vi "_IRR_mkpk.vi"(0 "Bias_LO_equip":T4={"Node address"=19, "CAN Interface"="CAN0", "Cartridge band"=10, "Slave Node in"={"Address"=19, "Serial Number"=[16, -88, -112, 75, 1, 8, 0, 24]}, "ObjHandle out"=93192256, "POL"=0, "sb"=1, "GPIB_SM (SIS S,V)"="24", "GPIB_DMM (SIS I)"="22", "GPIB_SM (MAG I) "="25", "GPIB_SG(LO)"="19", "GPIB_PW (PAMP) "="6", "GPIB_TMP1(8ch)"="12", "GPIB_TMP2(2ch)  "="13", "WCA_avg"=10, "Rsen"=10.0, "BiasModule"=1, "LOModule "=2, "WCA_LO_FREQ_SET"={"YTO Low freq. [GHz]"=14.66, "YTO High freq. [GHz]"=17.5, "Kvco"=1, "Lock Pol."=0, "SET LO FREQ"=88.77778, "Multiplier"=6.0, "YTO (HEX)"=197, "YTO ( FREQ)"=14.796625, "NULL PLL INTEGRATOR"=FALSE}} {"WCA_LO_FREQ_SET"."YTO ( FREQ)" min=25 max=150 step=0.0001 format="%.3f"; "WCA_LO_FREQ_SET"."Multiplier" min=3 max=6 step=3; "WCA_LO_FREQ_SET"."SET LO FREQ" min=25 max=150 step=0.0001 format="%.3f"; "WCA_LO_FREQ_SET"."Lock Pol." items=["Lower", "Upper"]; "WCA_LO_FREQ_SET"."Kvco" items=["7.5MHz/V", "15MHz/V"]; "WCA_LO_FREQ_SET"."YTO High freq. [GHz]" format="%.3f"; "WCA_LO_FREQ_SET"."YTO Low freq. [GHz]" format="%.3f"; "LOModule" items=["Manual Gunn+PAMP"=0, "PLL GUNN+PAMP"=5, "B10Lab LO"=1, "WCA LO"=2, ""=3, "YIG発信器"=4, "none"=99]; "BiasModule" items=["B10Lab Bias"=0, "WCA BiasModule"=1, "none"=99]; "Slave Node in"."Serial Number" format="%.0x"; "Slave Node in"."Address" format="%.0x"; "Cartridge band" max=10 step=1; "Node address" format="%.0x"}, 1 "Control":T8={"GPIB_ATT"="28", "6501Dev#"=1, "GPIB_SP"="18", "GPIB_PM"="13", "GPIB_DSA"="11", "GPIB_DMM (TPD)"="23", "GPIB_MPI"="COM9", "mortor設定"=[{"Axis"=0, "ID"=0, "HIspeed"=200.0, "LOspeed"=100.0, "ACCEL(ms)"=100.0, "Sratio"=50.0, "フリーラン\n"=FALSE, "文字列"="DSB HOT/COLD"}, {"Axis"=1, "ID"=0, "HIspeed"=4.0, "LOspeed"=4.0, "ACCEL(ms)"=100.0, "Sratio"=50.0, "フリーラン\n"=TRUE, "文字列"="SubMM Att"}, {"Axis"=0, "ID"=0, "HIspeed"=200.0, "LOspeed"=100.0, "ACCEL(ms)"=100.0, "Sratio"=50.0, "フリーラン\n"=FALSE, "文字列"="MPI Port1"}, {"Axis"=1, "ID"=0, "HIspeed"=200.0, "LOspeed"=100.0, "ACCEL(ms)"=100.0, "Sratio"=50.0, "フリーラン\n"=FALSE, "文字列"="MPI Port2"}, {"Axis"=1, "ID"=0, "HIspeed"=200.0, "LOspeed"=100.0, "ACCEL(ms)"=100.0, "Sratio"=50.0, "フリーラン\n"=TRUE, "文字列"="gainComp"}], "DATAパス"=path "C:/Documents and Settings/band10/デスクトップ/data/cartridge/CCA03/CCA-03-13/110831_etc", "mixer param file "=path "Z:/band10/Labview_ALMA/MIX95/test", "comment"="xttest", "ColdCarts"="003601", "Th"=299.0, "Tc"=77.0, "Set_SIS_volt"=2.1, "Offset"=0.0, "control"=0, "FreqLO"=799.0, "Set_Mag_Cur"=13.664233576642335, "MPI offset(mm)"=23.152, "HOT/COLD"=0} {"HOT/COLD" items=["DSB", "SBR (Cart.)", "GainComp", "SBR (MIX)"]; "control" items=["CLOSE LOOP", "OPEN LOOP", "Not Control"]}, 2 "CrossTalk_mkpk":T7={"save"=TRUE, "file_name"="xtk_799.00_120_xttest.csv", "IF start"=4.0, "IF stop"=12.0, "IF step"=1.0}, 3 "PAV配列":cluster{"VD":dbl, "VG ":dbl, "文字列":string}[](array[cluster])=[{"VD"=0.0, "VG "=-0.04, "文字列"="WCA P0"}, {"VD"=0.0, "VG "=-0.04, "文字列"="WCA P1"}, {"VD"=1.75, "VG "=2.1, "文字列"="B10 PAMP"}] {"VG" min=-1.0 max=4.0; "VD" min=0.0 max=2.5}, 4 "_LO_P_OPT":T3={"範囲配列"=[{"Start"=1.0, "Stop"=3.5, "Step"=0.01, "ｂｙ"="NEL VG"}, {"Start"=40.0, "Stop"=75.0, "Step"=1.0, "ｂｙ"="Motor"}, {"Start"=1.0, "Stop"=2.5, "Step"=0.1, "ｂｙ"="WCA VD"}], "Optimize"=0, "file_name"="LP_914.0_Tmin_100519.csv", "Save?"=FALSE, "measure"=2, "current(uA)"=60.0, "wait(ms)"=0, "IFfrq(GHz)"=8.0, "aveg"=10, "SISparam option"=2} {"SISparam option" items=["Volt and Current", "Volt only"]; "measure" items=["Pmax (only HOT)", "Tmin (HOT/COLD)", "C current"]; "Optimize" items=["Sweep", "黄金分割"]; "範囲配列"."Step" format="%.2f"; "範囲配列"."Stop" format="%.2f"; "範囲配列"."Start" format="%.2f"}) -> (7 "LOPopt P0":string="LOPt,799.00,1.46,1.88,38.10,0.00,0.00,0.00,2.10,,WCA,0.003815,4.013062,-0.021667,  1.030579,172.775269,-0.025177,")   [LabVIEW 2012]
uses:
  <vilib>/express/express arith-compare/Formula/XNode/ExpressFormulaBlockNode.xnode
panel:
  out "結果":string="4.000015,-97.540000,-93.196000,  -9.974000,-47.367000,-107.514000, -6.485000,-40.957000,-99.681000 , LOPt,799.00,1.46,1.88,38.19,0.00,0.00,0.00,2.19,,WCA,0.003662,3.952026,-0.022125,  1.031342,172.851562,-0.025787, ,LOPt,799.00,1.90,1.89,41.31,0.00,0.00,0.00,0.31,,WCA,1.335449,186.492920,-0.022125,  0.001831,3.158569,-0.025787, \n5.000041,-92.917000,-98.660000,  -10.003000,-45.366000,-102.920000, -7.055000,-44.960000,-105.715000 , LOPt,799.00,1.46,1.88,36.93,0.00,0.00,0.00,0.93,,WCA,0.003510,4.043579,-0.022736,  1.030426,172.744751,-0.025635, ,LOPt,799.00,1.90,1.90,41.12,0.00,0.00,0.00,0.12,,WCA,1.335754,186.691284,-0.021820,  0.001984,3.265381,-0.025330, \n6.000013,-94.024000,-94.568000,  -8.711000,-43.164000,-102.735000, -5.761000,-42.975000,-100.329000 , LOPt,799.00,1.46,1.87,37.45,0.00,0.00,0.00,1.45,,WCA,0.003510,3.936768,-0.022278,  1.030579,172.760010,-0.025940, ,LOPt,799.00,1.90,1.89,41.11,0.00,0.00,0.00,0.11,,WCA,1.336365,186.798096,-0.022736,  0.001831,3.173828,-0.025940, \n"
  out "XYグラフ":cluster{dbl[], dbl[]}[](graph)=[{[4.000015156, 5.000041231, 6.000013312], [-97.53999999999999, -92.917, -94.024]}, {[4.000015156, 5.000041231, 6.000013312], [-93.196, -98.66, -94.568]}]
  out "LOPopt P1":string="LOPt,799.00,1.90,1.89,41.11,0.00,0.00,0.00,0.11,,WCA,1.336365,186.798096,-0.022736,  0.001831,3.173828,-0.025940,"
  out "crossTK P1":dbl=-100.329 format="%#_6p"
  out "xpol P1":dbl=-42.975 format="%#_6p"
  out "copol P1":dbl=-5.761 format="%#_6p"
  in  "SP_set":T1={"start(GHz)"=3.5, "stop(GHz) "=12.5, "BW(MHz)"=0.0001, "VBW(Hz)"=30.0, "ref(dBm)"=0.0, "log(dB)"=15.0, "AVEG"=30, "AVEG ON/OFF"=FALSE, "Auto Align ON/OFF"=FALSE, "GPIB"="18", "point"=801}
  in  "IFBOX":T2={" Output"=1, "YIG Fc(GHz)"=4.0, " Filter"=3, "Input"=1} {"Input" items=["1:Pol 0"=1, "2:Pol 1"=2, "3:dummy"=3, "4:NoiseSource"=4]; "Filter" items=["1:YIG"=1, "2:direct"=2, "3:4-12BPF"=3, "4:direct 4-12BPF"=4]; "Output" items=["1:Speana"=1, "2:PowerMeter"=2, "3:dummy"=3, "4:TPD"=4]}
  in  "RF":T5={"RF(GHz)"=800.0, "mm_multi(4or6)"=6.0, "SGPOUT(dBm)"=10.0, "SGGPIB"="29", "PAMP GPIB"="6", "VD (V)"=1.7, "VG (V)"=2.2, "multi (V)"=8.0} {"multi (V)" min=0.0 max=15.0 step=0.5; "VG (V)" min=0.0 max=4.0 step=0.1; "VD (V)" min=0.0 max=1.85 step=0.1}
  out "crossTK P0":dbl=-102.735 format="%#_6p"
  out "xpol P0":dbl=-43.164 format="%#_6p"
  out "copol P0":dbl=-8.711 format="%#_6p"
  out "frq":dbl=6.000013312 format="%#_6p"
  in  "SIS_Deflux_heater":T6={"ON開始時間（mｓ）"=3000.0, "ON継続時間（mｓ）"=1000.0, "測定終了時間（mｓ）"=60000.0, "SIS Volt（mV)"=0.5, "GPIB_PW (SISHeater) "="3", "SAVE"=TRUE}
  out "初期時間（s）":dbl=3379641043.615625
  # "LO freq. [GHz]"
  # "YTO LOW\n/High Freq."
  # "ZERO Intgrtr"
  # "Node Address"
  # "Serial Number"
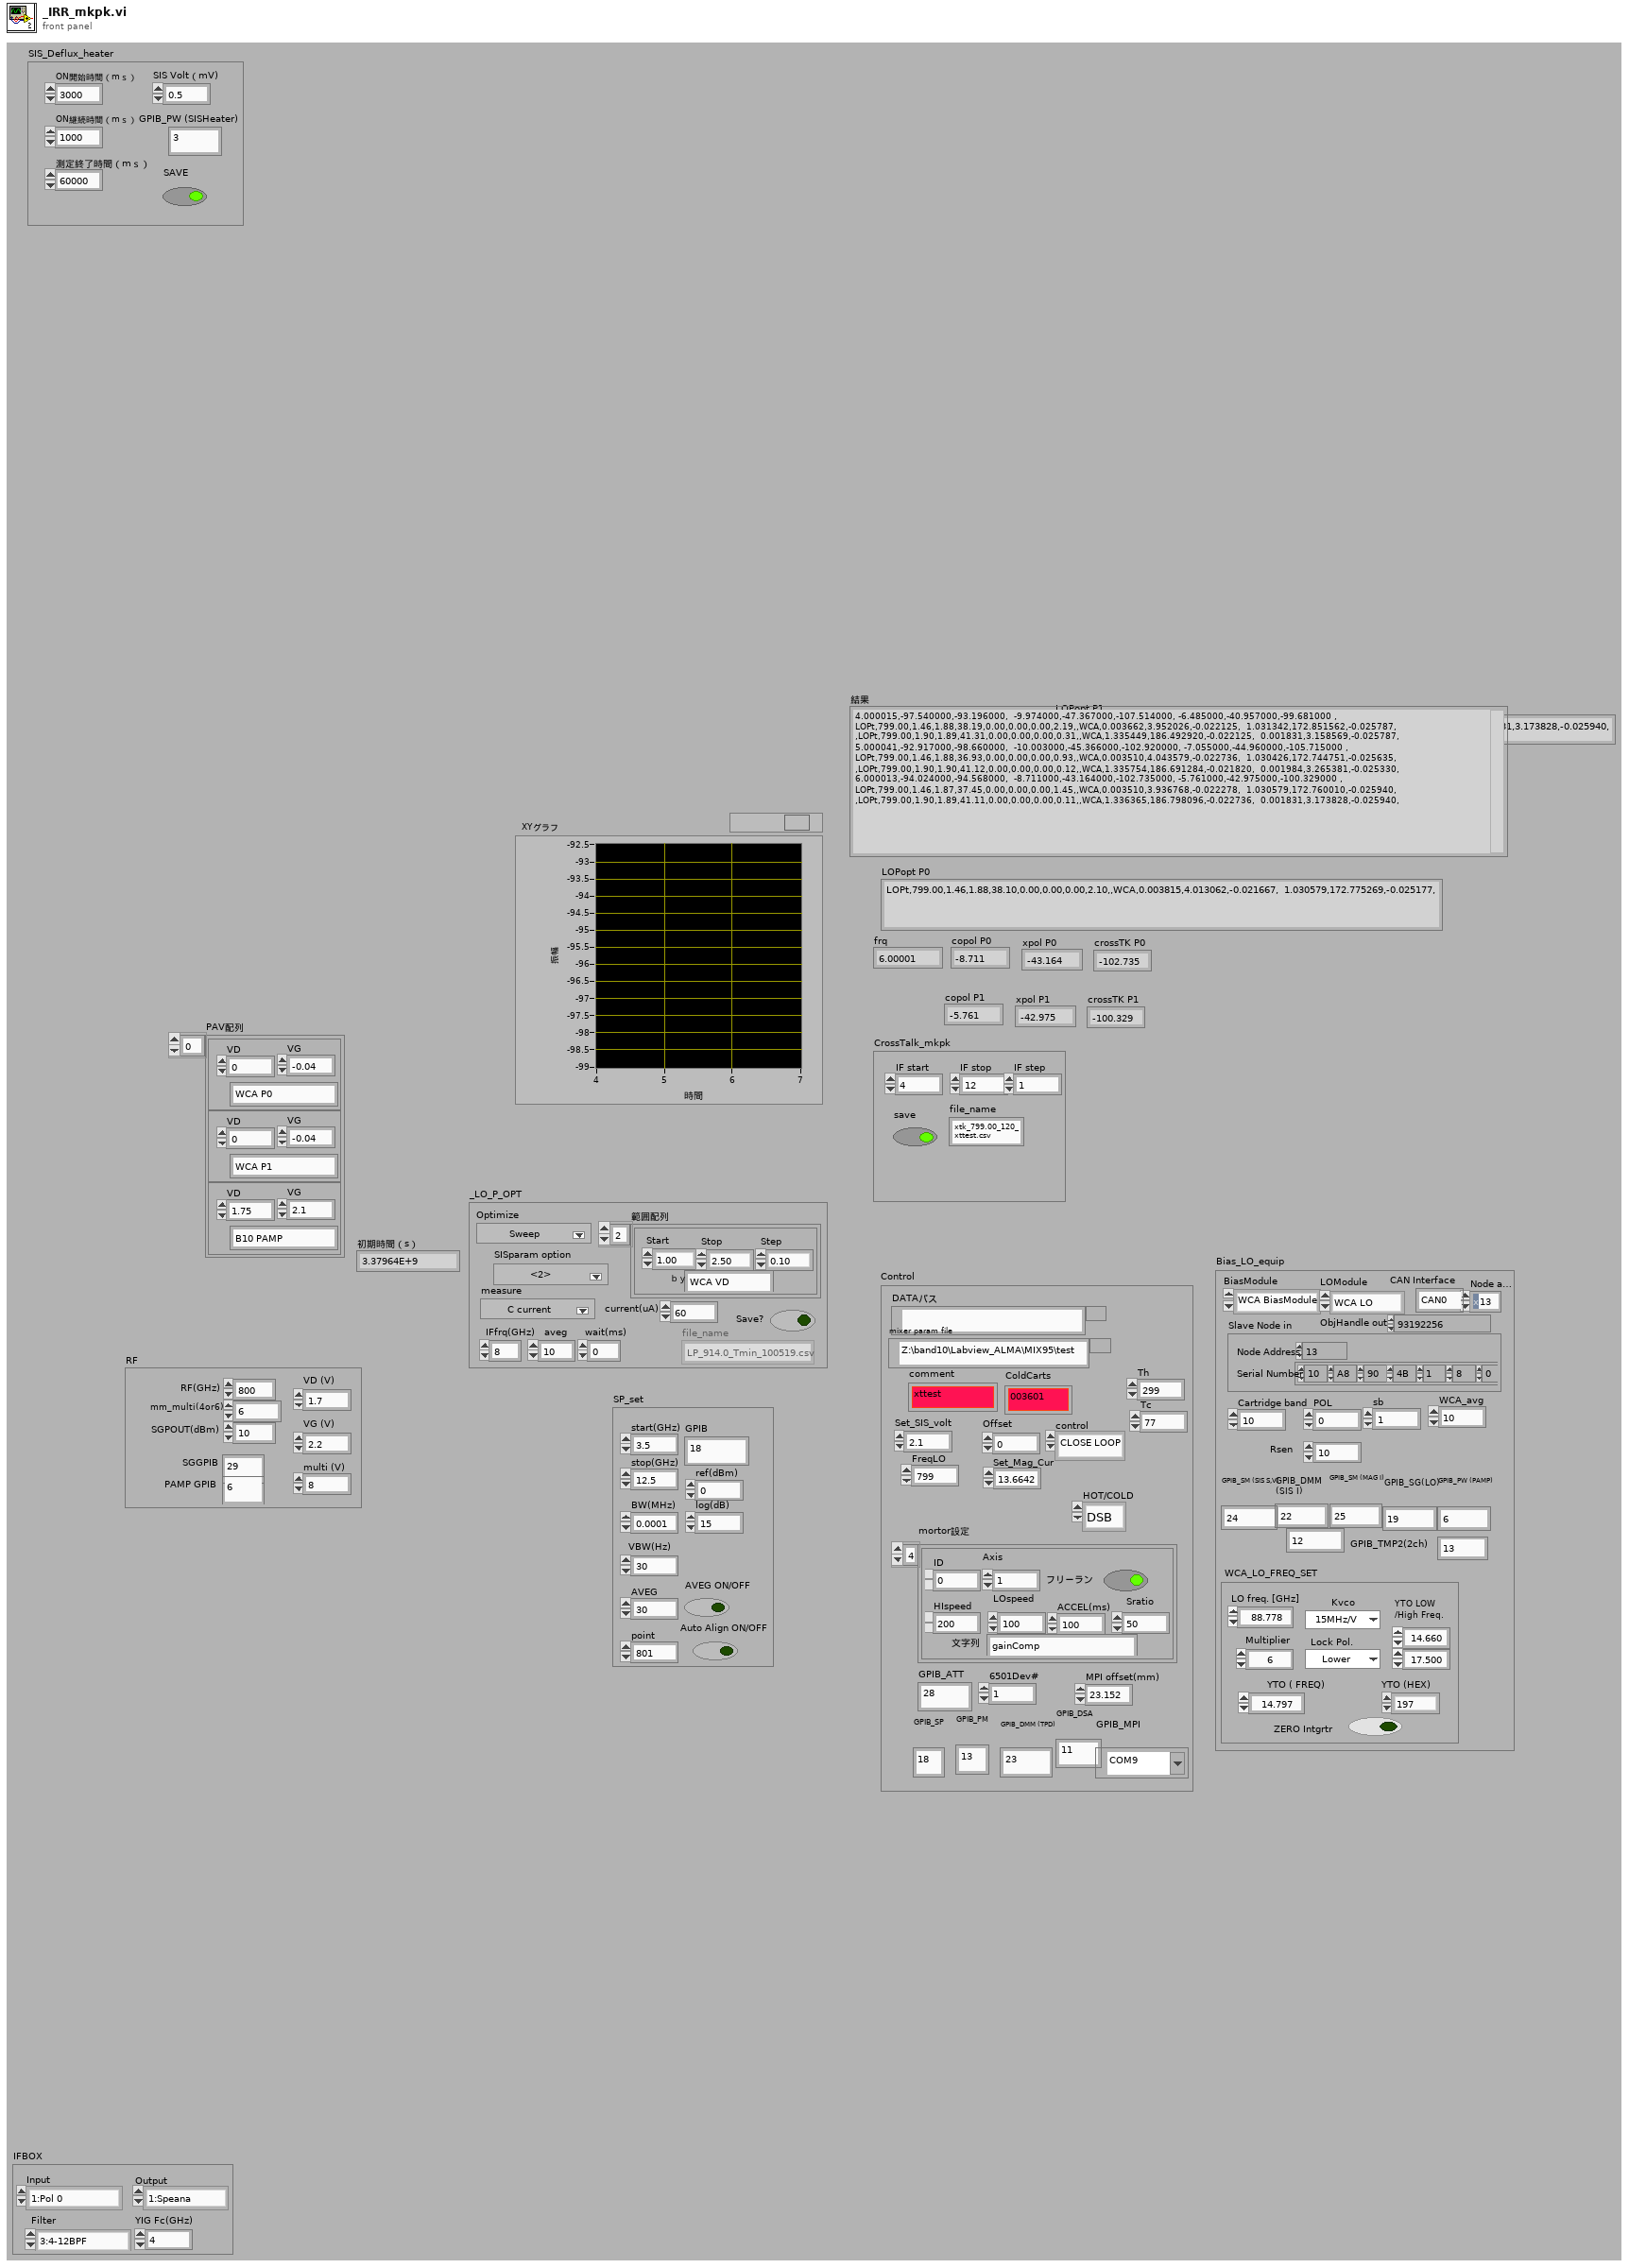
[diagram p1: front panel]
types:
  T1 = cluster{"start(GHz)":dbl, "stop(GHz) ":dbl, "BW(MHz)":dbl, "VBW(Hz)":dbl, "ref(dBm)":dbl, "log(dB)":dbl, "AVEG":i16, "AVEG ON/OFF":bool, "Auto Align ON/OFF":bool, "GPIB":string, "point":i16}
  T2 = cluster{" Output":u16, "YIG Fc(GHz)":dbl, " Filter":u16, "Input":u16}
  T3 = cluster{"範囲配列":cluster{"Start":dbl, "Stop":dbl, "Step":dbl, "ｂｙ":string}[], "Optimize":u16, "file_name":string, "Save?":bool, "measure":u16, "current(uA)":dbl, "wait(ms)":i32, "IFfrq(GHz)":dbl, "aveg":i32, "SISparam option":u16}
  T4 = cluster{"Node address":u16, "CAN Interface":string, "Cartridge band":u32, "Slave Node in":cluster{"Address":i16, "Serial Number":i8[]}, "ObjHandle out":u32, "POL":u32, "sb":u32, "GPIB_SM (SIS S,V)":string, "GPIB_DMM (SIS I)":string, "GPIB_SM (MAG I) ":string, "GPIB_SG(LO)":string, "GPIB_PW (PAMP) ":string, "GPIB_TMP1(8ch)":string, "GPIB_TMP2(2ch)  ":string, "WCA_avg":i32, "Rsen":dbl, "BiasModule":u16, "LOModule ":u16, "WCA_LO_FREQ_SET":cluster{"YTO Low freq. [GHz]":sgl, "YTO High freq. [GHz]":sgl, "Kvco":u16, "Lock Pol.":u16, "SET LO FREQ":sgl, "Multiplier":sgl, "YTO (HEX)":u16, "YTO ( FREQ)":sgl, "NULL PLL INTEGRATOR":bool}}
  T5 = cluster{"RF(GHz)":dbl, "mm_multi(4or6)":dbl, "SGPOUT(dBm)":dbl, "SGGPIB":string, "PAMP GPIB":string, "VD (V)":dbl, "VG (V)":dbl, "multi (V)":dbl}
  T6 = cluster{"ON開始時間（mｓ）":dbl, "ON継続時間（mｓ）":dbl, "測定終了時間（mｓ）":dbl, "SIS Volt（mV)":dbl, "GPIB_PW (SISHeater) ":string, "SAVE":bool}
  T7 = cluster{"save":bool, "file_name":string, "IF start":dbl, "IF stop":dbl, "IF step":dbl}
  T8 = cluster{"GPIB_ATT":string, "6501Dev#":i16, "GPIB_SP":string, "GPIB_PM":string, "GPIB_DSA":string, "GPIB_DMM (TPD)":string, "GPIB_MPI":refnum<visa-resource-name>, "mortor設定":cluster{"Axis":i16, "ID":i16, "HIspeed":dbl, "LOspeed":dbl, "ACCEL(ms)":dbl, "Sratio":dbl, "フリーラン\n":bool, "文字列":string}[], "DATAパス":path, "mixer param file ":path, "comment":string, "ColdCarts":string, "Th":dbl, "Tc":dbl, "Set_SIS_volt":dbl, "Offset":dbl, "control":u16, "FreqLO":dbl, "Set_Mag_Cur":dbl, "MPI offset(mm)":dbl, "HOT/COLD":u16}
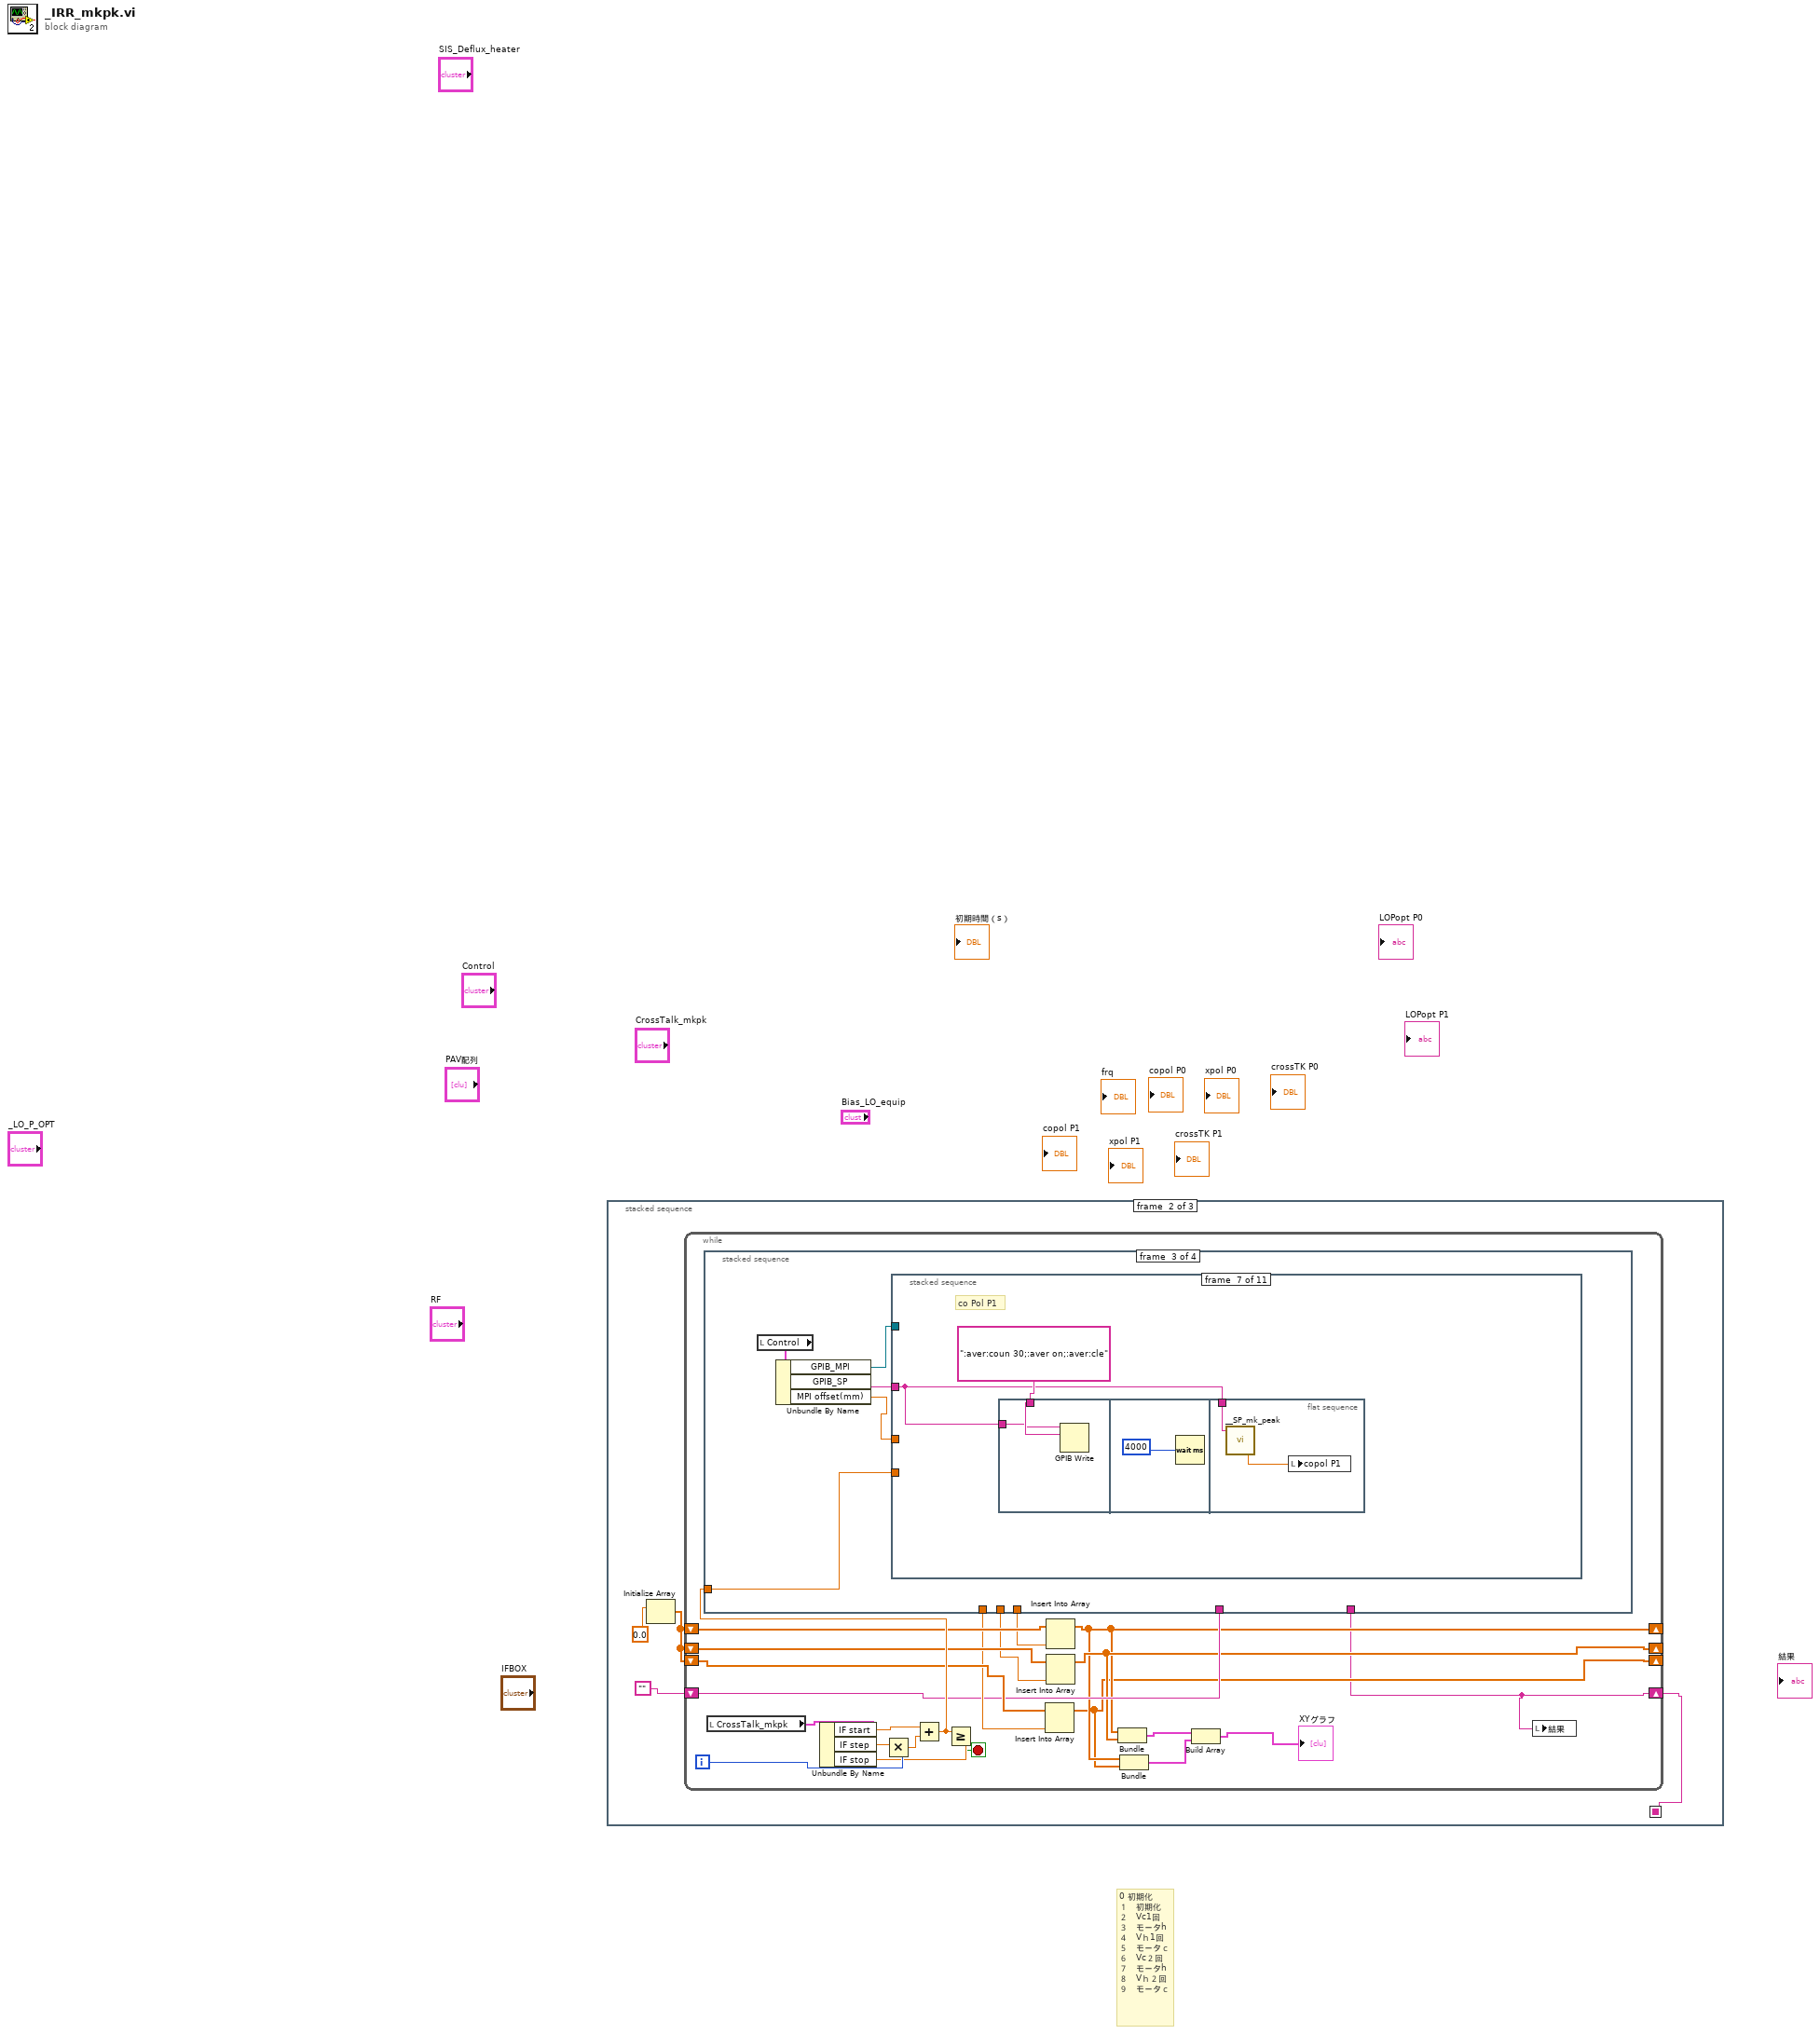
[diagram p0: block diagram]
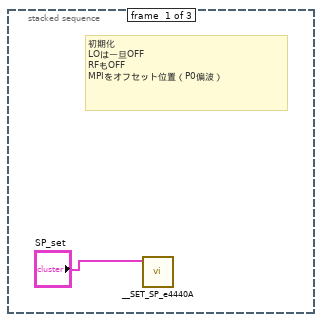
[diagram p2: hidden frame]
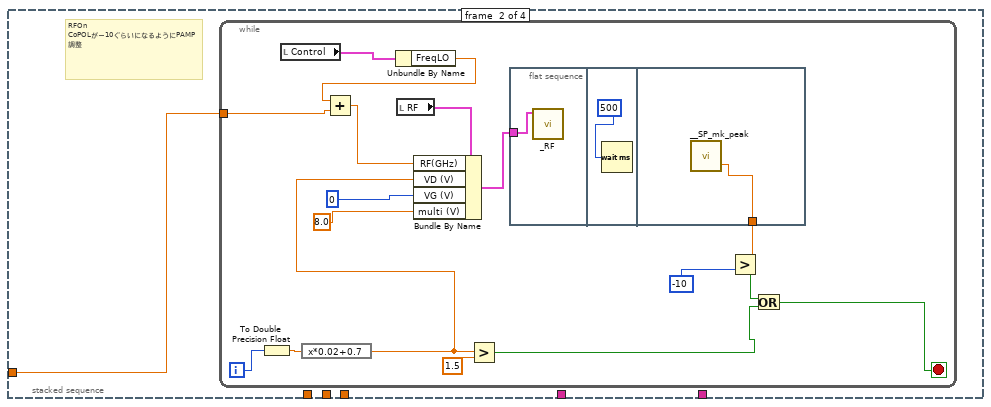
[diagram p4: hidden frame]
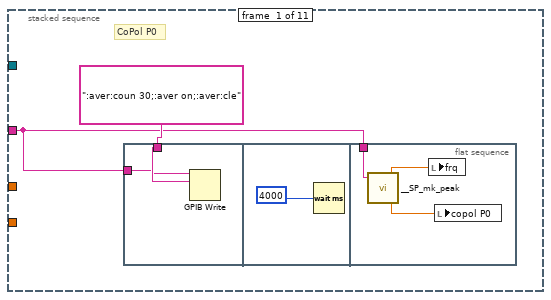
[diagram p5: hidden frame]
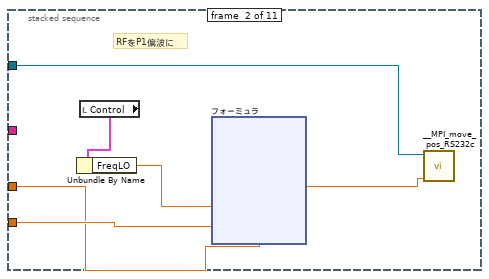
[diagram p6: hidden frame]
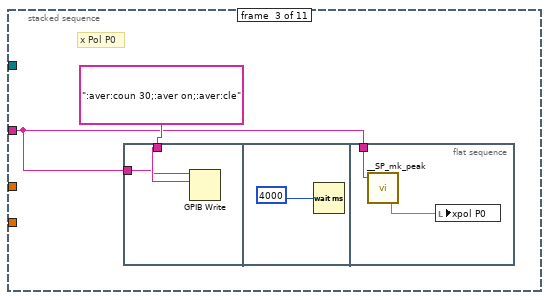
[diagram p7: hidden frame]
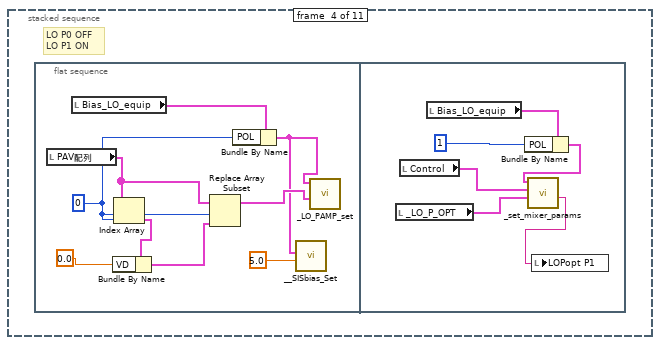
[diagram p8: hidden frame]
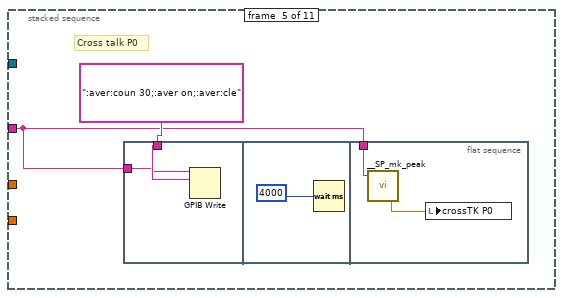
[diagram p9: hidden frame]
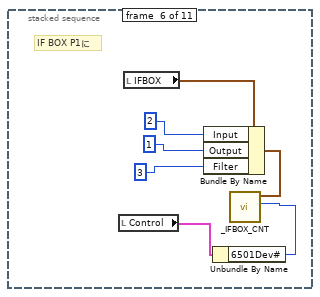
[diagram p10: hidden frame]
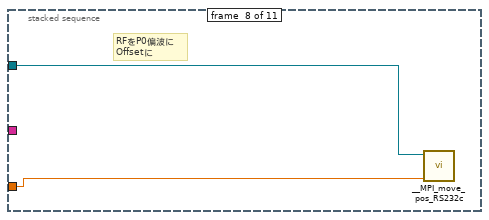
[diagram p11: hidden frame]
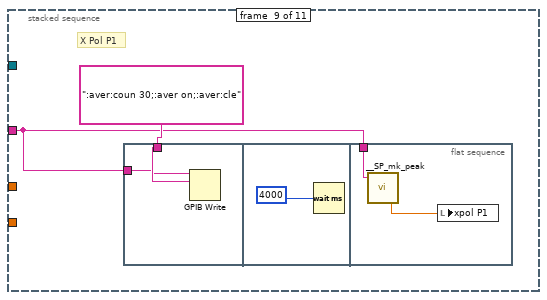
[diagram p12: hidden frame]
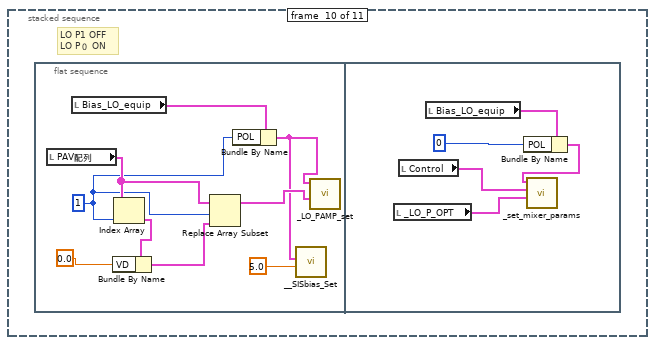
[diagram p13: hidden frame]
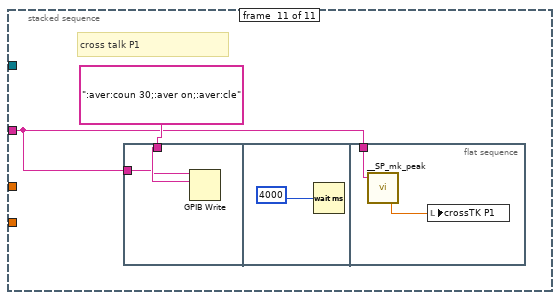
[diagram p14: hidden frame]
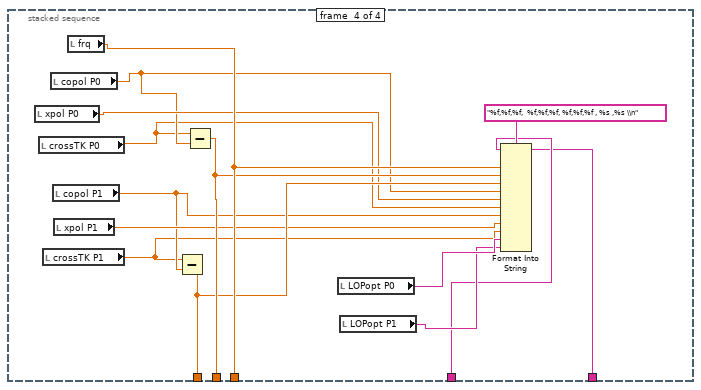
[diagram p15: hidden frame]
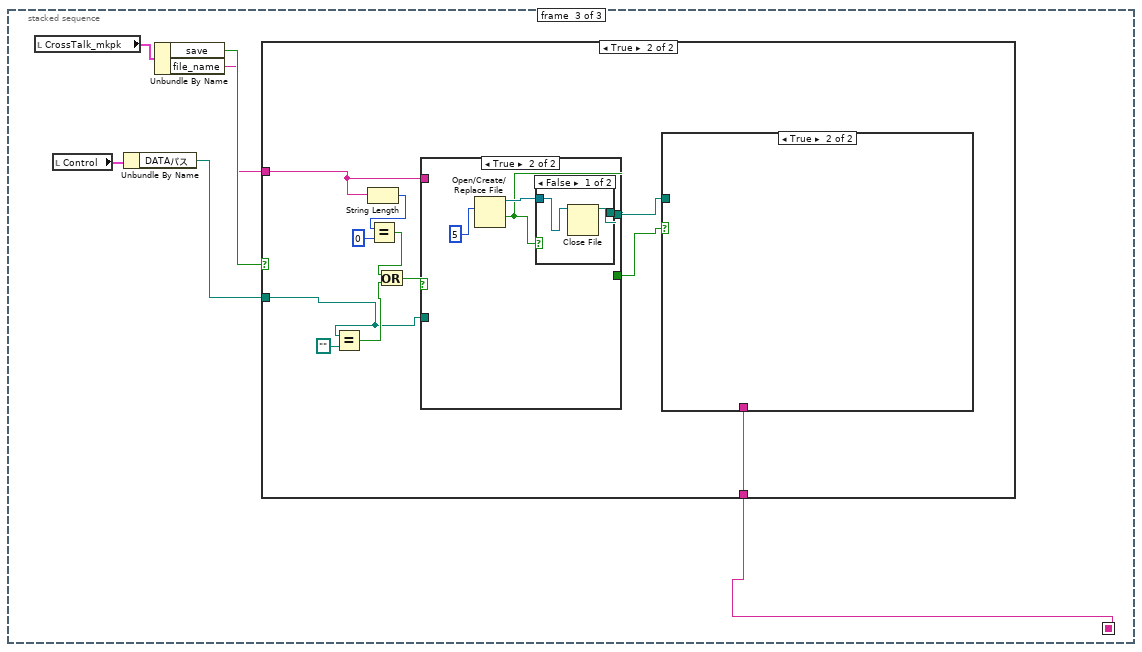
[diagram p16: hidden frame]
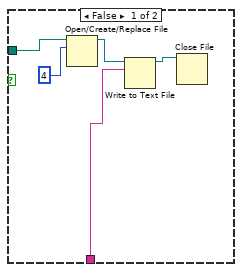
[diagram p18: hidden frame]
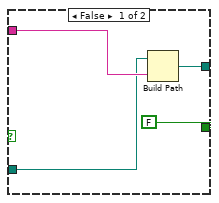
[diagram p19: hidden frame]
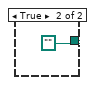
[diagram p20: hidden frame]
diagram:
  # "0 初期化\n１　初期化\n２　Vc1回\n３　モータh\n４　Vｈ1回\n５　モータｃ\n６　Vc２回\n７　モータh\n８　Vｈ２回\n９　モータｃ"
  n1 = stacked-sequence {
    seq-local: [_ w2 _] -> [_ _ w167]
    frame #0 {
      # "初期化\nLOは一旦OFF\nRFもOFF\nMPIをオフセット位置（P0偏波）"
      n2 = call "__SET_SP_e4440A.vi"("SP"="SP_set") -> ()  [unwired: 7 in]
    }
    frame #1 {
      n3 = Initialize Array(0.0) -> (w4:dbl[])  [unwired: 1 in]
      n4 = while {
        shift-right: [w11] -> _
        shift-left: w4 -> [w19]
        shift-right: [w12] -> _
        shift-left: w4 -> [w17]
        shift-right: [w10] -> _
        shift-left: w4 -> [w15]
        shift-right: [w6] -> w2
        shift-left: "" -> [w13]
        i -> [w25]
        stop <- w21 stop-if-true
        n5 = local read "CrossTalk_mkpk"() -> (w27:T7)
        n6 = Unbundle By Name(w27) -> ("IF start"=w24:dbl, "IF step"=w26:dbl, "IF stop"=w22:dbl)
        n7 = Multiply(x=w26, y=w25) -> (x*y=w23:dbl)
        n8 = Add(x=w24, y=w23) -> (x+y=w20:dbl)
        n9 = stacked-sequence {
          tunnel: w20 -> [_ w28 w51 _]
          tunnel: [_ _ _ w165] -> w18
          tunnel: [_ _ _ w164] -> w16
          tunnel: [_ _ _ w163] -> w14
          tunnel: w13 -> [_ _ _ w158]
          tunnel: [_ _ _ w157] -> w6
          frame #0 {
            # "P0 LO Set\nIFBOXをP0　SPにSet"
          }
          frame #1 {
            # "RFOn\nCoPOLがー10ぐらいになるようにPAMP調整"
            n10 = while {
              tunnel: w28 -> [w29]
              i -> [w45]
              stop <- w33 stop-if-true
              n11 = To Double Precision Float(number=w45) -> (double precision float=w44:dbl)
              n12 = local read "Control"() -> (w32:T8)
              n13 = expression code="x*0.02+0.7"(w44) -> (w40:dbl)
              n14 = Unbundle By Name(w32) -> ("FreqLO"=w30:dbl)
              n15 = Add(x=w30, y=w29) -> (x+y=w31:dbl)
              n16 = local read "RF"() -> (w42:T5)
              n17 = Bundle By Name(cluster=w42, "RF(GHz)"=w31, "VD (V)"=w40, "VG (V)"=0, "multi (V)"=8.0) -> (w41:T5)
              n18 = Greater?(x=w40, y=1.5) -> (0:w34:bool)
              n19 = flat-sequence {
                tunnel: w41 -> [w46]
                tunnel: [w48] -> w37
                frame #0 {
                  n20 = call "_RF.vi"("RF"=w46) -> ()  [unwired: 11 in]
                }
                frame #1 {
                  n21 = Wait (ms)(milliseconds to wait=500) -> ()  [unwired: 1 out]
                }
                frame #2 {
                  n22 = call "__SP_mk_peak.vi"() -> ("pow out"=w48:dbl)  [unwired: 3 in, 1 out]
                }
              }
              n23 = Greater?(x=w37, y=-10) -> (0:w35:bool)
              n24 = Or(x=w35, y=w34) -> (x .or. y?=w33:bool)
            }
          }
          frame #2 {
            n25 = local read "Control"() -> (w53:T8)
            n26 = Unbundle By Name(w53) -> ("GPIB_MPI"=w49:refnum<visa-resource-name>, "GPIB_SP"=w52:string, "MPI offset(mm)"=w50:dbl)
            n27 = stacked-sequence {
              tunnel: w52 -> [w54 _ w80 _ w102 _ w116 _ w125 _ w146]
              tunnel: w51 -> [_ w65 _ _ _ _ _ _ _ _ _]
              tunnel: w50 -> [_ w64 _ _ _ _ _ w123 _ _ _]
              tunnel: w49 -> [_ w63 _ _ _ _ _ w124 _ _ _]
              frame #0 {
                # "CoPol P0"
                n28 = flat-sequence {
                  tunnel: ":aver:coun 30;:aver on;:aver:cle" -> [w57]
                  tunnel: w54 -> [w56]
                  tunnel: w54 -> [w59]
                  frame #0 {
                    n29 = GPIB Write(0:w56, 1:w57) -> ()  [unwired: 3 in, 2 out]
                  }
                  frame #1 {
                    n30 = Wait (ms)(milliseconds to wait=4000) -> ()  [unwired: 1 out]
                  }
                  frame #2 {
                    n31 = call "__SP_mk_peak.vi"("GIPB番号"=w59) -> ("pow out"=w60:dbl, "Freq out"=w61:dbl)  [unwired: 2 in]
                    n32 = local write "frq"(w61) -> ()
                    n33 = local write "copol P0"(w60) -> ()
                  }
                }
              }
              frame #1 {
                # "RFをP1偏波に"
                n34 = local read "Control"() -> (w67:T8)
                n35 = Unbundle By Name(w67) -> ("FreqLO"=w66:dbl)
                n36 = xnode "フォーミュラ"("LO"=w66, "IF"=w65, "offset"=w64) -> ("結果"=w62:dbl)  [unwired: 1 in, 1 out]
                n37 = call "__MPI_move_pos_RS232c.vi"("pos"=w62, "VISAリソース名"=w63) -> ()  [unwired: 5 in, 1 out]
              }
              frame #2 {
                # "x Pol P0"
                n38 = flat-sequence {
                  tunnel: ":aver:coun 30;:aver on;:aver:cle" -> [w83]
                  tunnel: w80 -> [w82]
                  tunnel: w80 -> [w85]
                  frame #0 {
                    n39 = GPIB Write(0:w82, 1:w83) -> ()  [unwired: 3 in, 2 out]
                  }
                  frame #1 {
                    n40 = Wait (ms)(milliseconds to wait=4000) -> ()  [unwired: 1 out]
                  }
                  frame #2 {
                    n41 = call "__SP_mk_peak.vi"("GIPB番号"=w85) -> ("pow out"=w86:dbl)  [unwired: 2 in, 1 out]
                    n42 = local write "xpol P0"(w86) -> ()
                  }
                }
              }
              frame #3 {
                # "LO P0 OFF\nLO P1 ON"
                n43 = flat-sequence {
                  frame #0 {
                    w89 = 0
                    n44 = local read "PAV配列"() -> (w91:cluster{"VD":dbl, "VG ":dbl, "文字列":string}[])
                    n45 = local read "Bias_LO_equip"() -> (w90:T4)
                    n46 = Index Array(array=w91, index=w89) -> (element=w94:cluster{"VD":dbl, "VG ":dbl, "文字列":string})
                    n47 = Bundle By Name(cluster=w94, "VD"=0.0) -> (w95:cluster{"VD":dbl, "VG ":dbl, "文字列":string})
                    n48 = Replace Array Subset(array=w91, new element=w95, index=w89) -> (w93:cluster{"VD":dbl, "VG ":dbl, "文字列":string}[])
                    n49 = Bundle By Name(cluster=w90, "POL"=w89) -> (w88:T4)
                    n50 = call "__SISbias_Set.vi"("Set_V"=5.0, "Bias_LO_equip"=w88) -> ()  [unwired: 9 in, 1 out]
                    n51 = call "_LO_PAMP_set.vi"("PAV配列"=w93, "Bias_LO_equip"=w88) -> ()  [unwired: 10 in]
                  }
                  frame #1 {
                    n52 = local read "_LO_P_OPT"() -> (w101:T3)
                    n53 = local read "Control"() -> (w96:T8)
                    n54 = local read "Bias_LO_equip"() -> (w100:T4)
                    n55 = Bundle By Name(cluster=w100, "POL"=1) -> (w98:T4)
                    n56 = call "_set_mixer_params.vi"("_LO_P_OPT"=w101, "Control"=w96, "Bias_LO_equip"=w98) -> ("文字列"=w97:string)  [unwired: 6 in, 2 out]
                    n57 = local write "LOPopt P1"(w97) -> ()
                  }
                }
              }
              frame #4 {
                # "Cross talk P0"
                n58 = flat-sequence {
                  tunnel: ":aver:coun 30;:aver on;:aver:cle" -> [w105]
                  tunnel: w102 -> [w104]
                  tunnel: w102 -> [w107]
                  frame #0 {
                    n59 = GPIB Write(0:w104, 1:w105) -> ()  [unwired: 3 in, 2 out]
                  }
                  frame #1 {
                    n60 = Wait (ms)(milliseconds to wait=4000) -> ()  [unwired: 1 out]
                  }
                  frame #2 {
                    n61 = call "__SP_mk_peak.vi"("GIPB番号"=w107) -> ("pow out"=w108:dbl)  [unwired: 2 in, 1 out]
                    n62 = local write "crossTK P0"(w108) -> ()
                  }
                }
              }
              frame #5 {
                # "IF BOX P1に"
                n63 = local read "Control"() -> (w114:T8)
                n64 = local read "IFBOX"() -> (w113:T2)
                n65 = Bundle By Name(cluster=w113, "Input"=2, "Output"=1, "Filter"=3) -> (w112:T2)
                n66 = Unbundle By Name(w114) -> ("6501Dev#"=w115:i16)
                n67 = call "_IFBOX_CNT.vi"("6501Dev#"=w115, "IFBOX"=w112) -> ()  [unwired: 6 in]
              }
              frame #6 {
                # "co Pol P1"
                n68 = flat-sequence {
                  tunnel: ":aver:coun 30;:aver on;:aver:cle" -> [w119]
                  tunnel: w116 -> [w118]
                  tunnel: w116 -> [w121]
                  frame #0 {
                    n69 = GPIB Write(0:w118, 1:w119) -> ()  [unwired: 3 in, 2 out]
                  }
                  frame #1 {
                    n70 = Wait (ms)(milliseconds to wait=4000) -> ()  [unwired: 1 out]
                  }
                  frame #2 {
                    n71 = call "__SP_mk_peak.vi"("GIPB番号"=w121) -> ("pow out"=w122:dbl)  [unwired: 2 in, 1 out]
                    n72 = local write "copol P1"(w122) -> ()
                  }
                }
              }
              frame #7 {
                # "RFをP0偏波に\nOffsetに"
                n73 = call "__MPI_move_pos_RS232c.vi"("pos"=w123, "VISAリソース名"=w124) -> ()  [unwired: 5 in, 1 out]
              }
              frame #8 {
                # "X Pol P1"
                n74 = flat-sequence {
                  tunnel: ":aver:coun 30;:aver on;:aver:cle" -> [w128]
                  tunnel: w125 -> [w127]
                  tunnel: w125 -> [w130]
                  frame #0 {
                    n75 = GPIB Write(0:w127, 1:w128) -> ()  [unwired: 3 in, 2 out]
                  }
                  frame #1 {
                    n76 = Wait (ms)(milliseconds to wait=4000) -> ()  [unwired: 1 out]
                  }
                  frame #2 {
                    n77 = call "__SP_mk_peak.vi"("GIPB番号"=w130) -> ("pow out"=w131:dbl)  [unwired: 2 in, 1 out]
                    n78 = local write "xpol P1"(w131) -> ()
                  }
                }
              }
              frame #9 {
                # "LO P1 OFF\nLO P０ ON"
                n79 = flat-sequence {
                  frame #0 {
                    w134 = 1
                    n80 = local read "PAV配列"() -> (w136:cluster{"VD":dbl, "VG ":dbl, "文字列":string}[])
                    n81 = local read "Bias_LO_equip"() -> (w135:T4)
                    n82 = Index Array(array=w136, index=w134) -> (element=w139:cluster{"VD":dbl, "VG ":dbl, "文字列":string})
                    n83 = Bundle By Name(cluster=w139, "VD"=0.0) -> (w140:cluster{"VD":dbl, "VG ":dbl, "文字列":string})
                    n84 = Replace Array Subset(array=w136, new element=w140, index=w134) -> (w138:cluster{"VD":dbl, "VG ":dbl, "文字列":string}[])
                    n85 = Bundle By Name(cluster=w135, "POL"=w134) -> (w132:T4)
                    n86 = call "__SISbias_Set.vi"("Set_V"=5.0, "Bias_LO_equip"=w132) -> ()  [unwired: 9 in, 1 out]
                    n87 = call "_LO_PAMP_set.vi"("PAV配列"=w138, "Bias_LO_equip"=w132) -> ()  [unwired: 10 in]
                  }
                  frame #1 {
                    n88 = local read "_LO_P_OPT"() -> (w145:T3)
                    n89 = local read "Control"() -> (w141:T8)
                    n90 = local read "Bias_LO_equip"() -> (w144:T4)
                    n91 = Bundle By Name(cluster=w144, "POL"=0) -> (w142:T4)
                    n92 = call "_set_mixer_params.vi"("_LO_P_OPT"=w145, "Control"=w141, "Bias_LO_equip"=w142) -> ()  [unwired: 6 in, 3 out]
                  }
                }
              }
              frame #10 {
                # "cross talk P1"
                n93 = flat-sequence {
                  tunnel: ":aver:coun 30;:aver on;:aver:cle" -> [w149]
                  tunnel: w146 -> [w148]
                  tunnel: w146 -> [w151]
                  frame #0 {
                    n94 = GPIB Write(0:w148, 1:w149) -> ()  [unwired: 3 in, 2 out]
                  }
                  frame #1 {
                    n95 = Wait (ms)(milliseconds to wait=4000) -> ()  [unwired: 1 out]
                  }
                  frame #2 {
                    n96 = call "__SP_mk_peak.vi"("GIPB番号"=w151) -> ("pow out"=w152:dbl)  [unwired: 2 in, 1 out]
                    n97 = local write "crossTK P1"(w152) -> ()
                  }
                }
              }
            }
          }
          frame #3 {
            n98 = local read "xpol P0"() -> (w162:dbl)
            n99 = local read "crossTK P0"() -> (w155:dbl)
            n100 = local read "crossTK P1"() -> (w153:dbl)
            n101 = local read "copol P0"() -> (w156:dbl)
            n102 = local read "copol P1"() -> (w154:dbl)
            n103 = local read "xpol P1"() -> (w161:dbl)
            n104 = local read "frq"() -> (w165:dbl)
            n105 = Subtract(x=w153, y=w154) -> (x-y=w163:dbl)
            n106 = Subtract(x=w155, y=w156) -> (x-y=w164:dbl)
            n107 = local read "LOPopt P0"() -> (w160:string)
            n108 = local read "LOPopt P1"() -> (w159:string)
            n109 = Format Into String(format string="%f,%f,%f,  %f,%f,%f, %f,%f,%f , %s ,%s \\n", initial string=w158, w165, w164, w163, w156, w162, w155, w154, w161, w153, w160, w159) -> (resulting string=w157:string)  [unwired: 1 in, 1 out]
          }
        }
        n110 = Greater Or Equal?(x=w20, y=w22) -> (x >= y?=w21:bool)
        n111 = Insert Into Array(array=w15, new element=w14) -> (w10:dbl[])  [unwired: 1 in]
        n112 = Insert Into Array(array=w19, new element=w18) -> (w11:dbl[])  [unwired: 1 in]
        n113 = Insert Into Array(array=w17, new element=w16) -> (w12:dbl[])  [unwired: 1 in]
        n114 = Bundle(w11, w12) -> (w9:cluster{dbl[], dbl[]})  [unwired: 1 in]
        n115 = Bundle(w11, w10) -> (w8:cluster{dbl[], dbl[]})  [unwired: 1 in]
        n116 = Build Array(w9, w8) -> (→"XYグラフ":cluster{dbl[], dbl[]}[])
        n117 = local write "結果"(w6) -> ()
      }
    }
    frame #2 {
      n118 = local read "CrossTalk_mkpk"() -> (w172:T7)
      n119 = local read "Control"() -> (w169:T8)
      n120 = Unbundle By Name(w169) -> ("DATAパス"=w168:path)
      n121 = Unbundle By Name(w172) -> ("save"=w171:bool, "file_name"=w170:string)
      n122 = case shown="TRUE" w171 {
        tunnel: w170 -> [_ w177]
        tunnel: w168 -> [_ w176]
        tunnel: w167 -> [_ w173]
        frame False {
        }
        frame True {
          n123 = Equal?(x=w176, y=path "") -> (x = y?=w178:bool)
          n124 = String Length(string=w177) -> (length=w183:i32)
          n125 = Equal?(x=w183, y=0) -> (x = y?=w179:bool)
          n126 = Or(x=w179, y=w178) -> (x .or. y?=w180:bool)
          n127 = case shown="TRUE" w180 {
            tunnel: w177 -> [w192 _]
            tunnel: [w191 w194] -> w175
            tunnel: [FALSE w193] -> w174
            tunnel: w176 -> [w189 _]
            frame False {
              n128 = Build Path(base path=w189, name or relative path=w192) -> (appended path=w191:path)
            }
            frame True {
              n129 = Open/Create/Replace File(operation (0:open)=5) -> (refnum out=w195:refnum<file>, cancelled=w193:bool)  [unwired: 5 in, 1 out]
              n130 = case shown="FALSE" w193 {
                tunnel: w195 -> [w198 _]
                tunnel: [w197 path ""] -> w194
                frame False {
                  n131 = Close File(refnum=w198) -> (path=w197:path)  [unwired: 1 in, 1 out]
                }
                frame True {
                }
              }
            }
          }
          n132 = case shown="TRUE" w174 {
            tunnel: w175 -> [w188 _]
            tunnel: w173 -> [w184 _]
            frame False {
              n133 = Open/Create/Replace File(file path (use dialog)=w188, operation (0:open)=4) -> (refnum out=w186:refnum<file>)  [unwired: 4 in, 2 out]
              n134 = Write to Text File(file (use dialog)=w186, text=w184) -> (refnum out=w185:refnum<file>)  [unwired: 2 in, 2 out]
              n135 = Close File(refnum=w185) -> ()  [unwired: 1 in, 2 out]
            }
            frame True {
            }
          }
        }
      }
    }
  }
